vi "Controlled voltage ramp checking current.vi"(6 "Barcodes in":string[](array[string]), 9 "Stop Program":bool, 11 "VISA Refnum in":refnum<visa-resource-name>) -> (0 "error out":errorcluster, 1 "channel 4 currents":dbl[](array[numeric]), 2 "channel 3 currents":dbl[](array[numeric]), 3 "channel 2 currents":dbl[](array[numeric]), 5 "channel 1 currents":dbl[](array[numeric]), 7 "BoardHandle out 2":T1, 10 "Power Supply Trip":bool)   [LabVIEW 2020]
uses:
  Program Files/National Instruments/LabVIEW 2018/instr.lib/CAEN PSM/CAEN PSM.lvlib
panel:
  out "Actual Voltage Level (V)":dbl format="%#_13g"
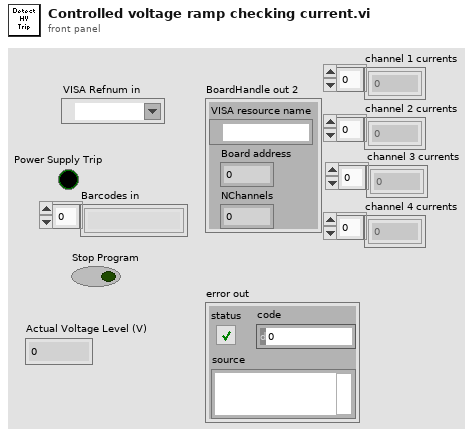
[diagram p1: front panel]
types:
  T1 = cluster{"VISA resource name":refnum<visa-resource-name>, "Board address":u8, "NChannels":u8}
  T2 = typedef "CAEN PSM.lvlib/BoardHandle.ctl" = cluster{"VISA resource name":refnum<visa-resource-name>, "Board address":u8, "NChannels":u8}
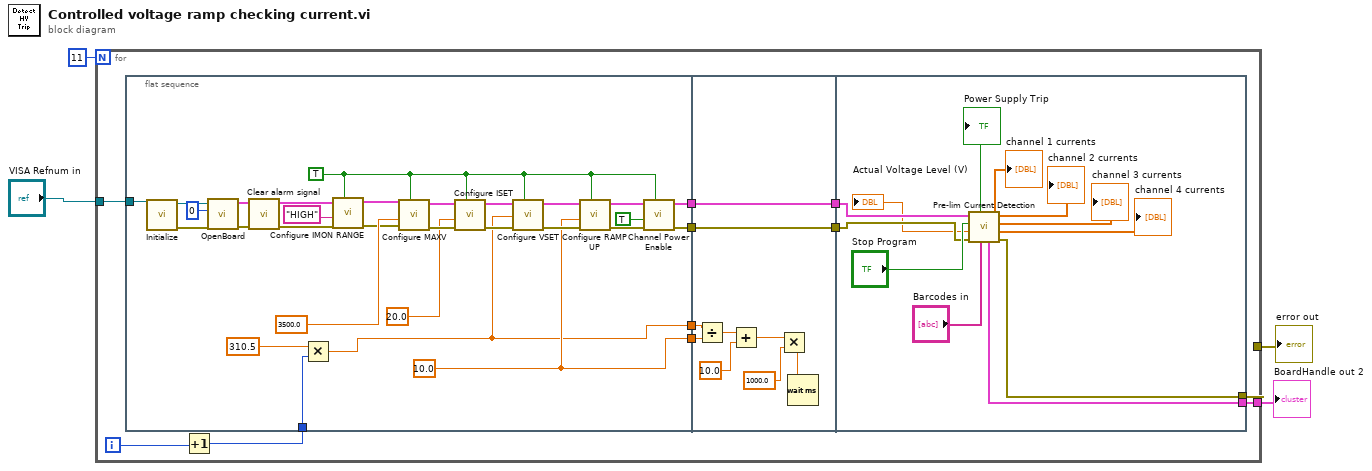
[diagram p0: block diagram]
diagram:
  n1 = for {
    N: 11 -> [_]
    tunnel: "VISA Refnum in" -> [w11]
    tunnel: [w10] -> w3
    tunnel: [w9] -> w2
    i -> [w6]
    n2 = flat-sequence {
      tunnel: [w18] -> w15
      tunnel: [w30] -> w14
      tunnel: [w29] -> w13
      tunnel: [w28] -> w12
      tunnel: w11 -> [w27]
      tunnel: w5 -> [w16]
      tunnel: w15 -> [w48]
      tunnel: w14 -> [w47]
      tunnel: w13 -> [w46]
      tunnel: w12 -> [w45]
      tunnel: [w46] -> w8
      tunnel: [w45] -> w7
      tunnel: [w62] -> w10
      tunnel: [w61] -> w9
      tunnel: w8 -> [w64]
      tunnel: w7 -> [w63]
      frame #0 {
        w20 = TRUE ("All Channels (F)")
        w30 = 10.0 ("Voltage Ramp Up (V/s)")
        n3 = call "Initialize.vi"("VISA resource name"=w27) -> ("error out"=w39:errorcluster, "VISA resource name out"=w36:refnum<visa-resource-name>)  [unwired: 9 in]
        n4 = call "OpenBoard.vi"("error in (no error)"=w39, "Board Address"=u8 0, "VISA resource name"=w36) -> ("error out"=w40:errorcluster, "BoardHandle"=w35:T2)  [unwired: 7 in]
        n5 = call "Clear alarm signal.vi"("error in (no error)"=w40, "BoardHandle"=w35) -> ("error out"=w25:errorcluster, "BoardHandle out"=w24:T2)  [unwired: 8 in]
        n6 = Multiply(x=310.5, y=w16) -> (x*y=w18:dbl)
        n7 = call "Configure IMON RANGE.vi"("All Channels (F)"=w20, "error in (no error)"=w25, "IMon range (LOW)"="HIGH", "BoardHandle"=w24) -> ("error out"=w21:errorcluster, "BoardHandle out"=w22:T2)  [unwired: 6 in]
        n8 = call "Configure MAXV.vi"("All Channels (F)"=w20, "error in (no error)"=w21, "Voltage Max (0.0 V)"=3500.0 ("VMax (Volts)"), "BoardHandle"=w22) -> ("error out"=w41:errorcluster, "BoardHandle out"=w34:T2)  [unwired: 6 in]
        n9 = call "Configure ISET.vi"("All Channels (F)"=w20, "error in (no error)"=w41, "Current Limit (0.00 uA)"=20.0 ("Current Limit (uA)"), "BoardHandle"=w34) -> ("error out"=w42:errorcluster, "BoardHandle out"=w33:T2)  [unwired: 6 in]
        n10 = call "Configure VSET.vi"("All Channels (F)"=w20, "error in (no error)"=w42, "Voltage Level (0.0 V)"=w18, "BoardHandle"=w33) -> ("error out"=w43:errorcluster, "BoardHandle out"=w32:T2)  [unwired: 6 in]
        n11 = call "Configure RAMP UP.vi"("All Channels (F)"=w20, "error in (no error)"=w43, "Voltage ramp up (0 V/s)"=w30, "BoardHandle"=w32) -> ("error out"=w44:errorcluster, "BoardHandle out"=w31:T2)  [unwired: 6 in]
        n12 = call "Channel Power Enable.vi"("All Channels (F)"=w20, "error in (no error)"=w44, "Enable (OFF)"=TRUE ("Boolean"), "BoardHandle"=w31) -> ("error out"=w28:errorcluster, "BoardHandle out"=w29:T2)  [unwired: 6 in]
      }
      frame #1 {
        n13 = Divide(x=w48, y=w47) -> (x/y=w51:dbl)
        n14 = Add(x=w51, y=10.0) -> (x+y=w52:dbl)
        n15 = Multiply(x=w52, y=1000.0) -> (x*y=w53:dbl)
        n16 = Wait (ms)(milliseconds to wait=w53) -> ()  [unwired: 1 out]
      }
      frame #2 {
        n17 = call "Pre-lim Current Detection.vi"("Barcodes in"="Barcodes in", "error in (no error)"=w63, "Stop Program"="Stop Program", "BoardHandle in"=w64) -> ("error out"=w62:errorcluster, "channel 4 currents"=→"channel 4 currents":dbl[], "channel 3 currents"=→"channel 3 currents":dbl[], "channel 2 currents"=→"channel 2 currents":dbl[], "BoardHandle out 3"=w61:T1, "channel 1 currents"=→"channel 1 currents":dbl[], "Power Supply Trip"=→"Power Supply Trip":bool, "Actual Voltage Level (V)"=→"Actual Voltage Level (V)":dbl)
      }
    }
    n18 = Increment(x=w6) -> (x+1=w5:i32)
  }
  "BoardHandle out 2" <- w2
  "error out" <- w3
